vi "generate_colour.vi"(4 "percentiles":T1, 6 "Colour":enum16{"Greyscale", "Colour"}(ring), 9 "image in":refnum<vi>) -> ()   [LabVIEW 2020]
uses:
  _controls/perc.ctl
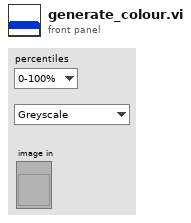
[diagram p1: front panel]
types:
  T1 = typedef "perc.ctl" = enum16{"0-100%", "0.1-0.99%", "1-99%", "5-95%", "10-90%", "20-80%"}
  T2 = typedef "cluster.range.sgl.ctl" = cluster{"min":sgl, "max":sgl}
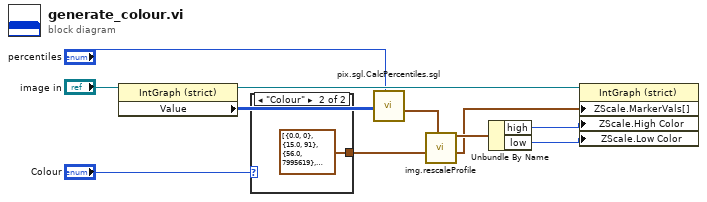
[diagram p0: block diagram]
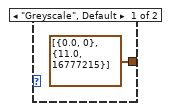
[diagram p2: hidden frame]
diagram:
  n1 = property class="IntGraph (strict)"(reference="image in") -> (reference out=w5:refnum<vi>, "Value"=w4:u16[][])  [unwired: 1 in, 1 out]
  n2 = case shown="\"Colour\"" "Colour" {
    tunnel: [cluster{dbl, u32}[] [{0.0, 0}, {11.0, 16777215}] ("MarkerVals in") cluster{dbl, u32}[] [{0.0, 0}, {15.0, 91}, {56.0, 7995619}, {96.0, 12779613}, {127.0, 15617024}, {144.0, 16741632}, {208.0, 16771584}, {224.0, 16777058}, {248.0, 16777215}, {255.0, 16777215}] ("MarkerValues")] -> w10
    frame "Greyscale", Default {
    }
    frame "Colour" {
    }
  }
  n3 = call "pix.sgl.CalcPercentiles.sgl.vi"("percentiles"="percentiles", "img in"=w4) -> ("range"=w9:T2)  [unwired: 9 in]
  n4 = call "img.rescaleProfile.vi"("range"=w9, "MarkerVals in (greyscale)"=w10) -> ("MarkerVals out"=w8:cluster{dbl, u32}[], "extrema"=w11:cluster{"high":u32, "low":u32})  [unwired: 8 out]
  n5 = Unbundle By Name(w11) -> ("high"=w7:u32, "low"=w6:u32)
  n6 = property class="IntGraph (strict)"(reference=w5, "ZScale.MarkerVals[]"=w8, "ZScale.High Color"=w7, "ZScale.Low Color"=w6) -> ()  [unwired: 1 in, 2 out]
